vi "CtrlHandlerNode.Python.vi"(0 "Diagram":refnum<vi>, 1 "Name":string, 2 "Ctrl":refnum<vi>, 3 "Type":T1=enum."Value Change", 4 "Data":variant) -> ()   [LabVIEW 2014]
uses:
  <vilib>/event_ctls.llb/lveventtype.ctl
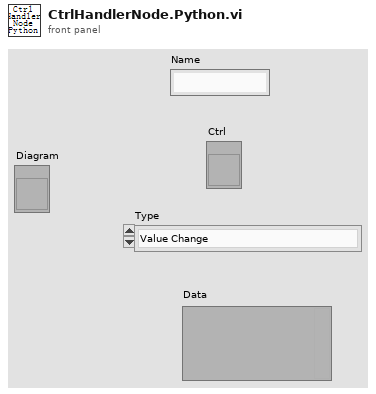
[diagram p1: front panel]
types:
  T1 = typedef "lveventtype.ctl" = enum32{"Null", "Timeout", "Annotation Menu Selection", "Annotation Menu Selection?", "App Instance Close", "App Instance Close?", "Autoscale Range Change", "Bookmark Info Change", "Cell Edit", "Cell Edit?", "Cursor Grab", "Cursor Grab?", "Cursor Menu Selection", "Cursor Menu Selection?", "Cursor Move", "Cursor Release", "Data Change", "Direction Change", "Display State Change", "Drag Ended", "Drag Enter", "Drag Leave", "Drag Over", "Drag Source Update", "Drag Starting", "Drag Starting?", "Drop", "Exec State Change", "Key Down", "Key Down?", "Key Repeat", "Key Repeat?", "Key Up", "Listbox Double Click", "Menu Activation?", "Menu Selection (App)", "Menu Selection? (App)", "Menu Selection (User)", "Mouse Down", "Mouse Down?", "Mouse Enter", "Mouse Leave", "Mouse Move", "Mouse Up", "Mouse Wheel", "NI Security User Change (App)", "Pane Size", "Panel Close", "Panel Close?", "Panel Resize", "Plot Attribute Change", "Scale Range Change", "Shortcut Menu Activation?", "Shortcut Menu Selection (App)", "Shortcut Menu Selection? (App)", "Shortcut Menu Selection (User)", "Tree Double Click", "Tree Drag", "Tree Drag?", "Tree Drop", "Tree Drop?", "Tree Item Close", "Tree Item Close?", "Tree Item Open", "Tree Item Open?", "User Event", "Value Change"}
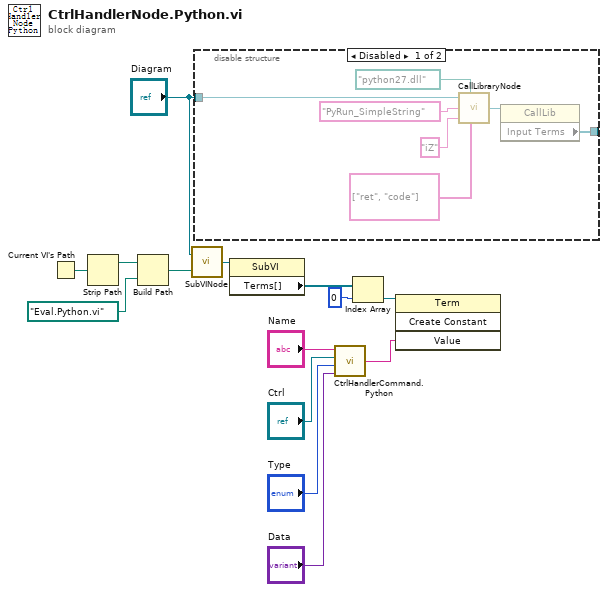
[diagram p0: block diagram]
diagram:
  n1 = Current VI's Path() -> (path=w6:path)
  n2 = Strip Path(path=w6) -> (stripped path=w5:path)  [unwired: 1 out]
  n3 = Build Path(base path=w5, name or relative path=path "Eval.Python.vi" ("Path")) -> (appended path=w3:path)
  n4 = call "SubVINode.vi"("Path"=w3, "Owner"="Diagram") -> ("Node"=w2:refnum<vi>)
  n5 = disable-structure shown="Disabled" {
    disable-tunnel: [w16 _] -> _
    disable-tunnel: "Diagram" -> [w15 _]
    frame Disabled {
      n6 = call "CallLibraryNode.vi"("Owner"=w15, "Library"=path "python27.dll" ("Library Path"), "Function"="PyRun_SimpleString" ("Function Name"), "Sig"="iZ", "Names"=string[] ["ret", "code"]) -> ("Node"=w17:refnum<vi>)
      n7 = property class="CallLib"(reference=w17) -> ("Input Terms"=w16:refnum<vi>[])  [unwired: 1 in, 2 out]
    }
    frame Enabled {
    }
  }
  n8 = property class="SubVI"(reference=w2) -> ("Terms[]"=w1:refnum<vi>[])  [unwired: 1 in, 2 out]
  n9 = call "CtrlHandlerCommand.Python.vi"("Data"="Data", "Type"="Type", "Ctrl"="Ctrl", "Name"="Name") -> ("Command"=w10:string)
  n10 = Index Array(array=w1, index=0) -> (element=w13:refnum<vi>)
  n11 = invoke class="Term" method="Create Constant"(reference=w13, "Value"=w10) -> ()  [unwired: 2 in, 4 out]
